vi "solar_cfg Read File (Var).vi"(0 "Config Path (*.ini)":path, 1 "Section (\"\" = Use Filename)":string, 2 "Comments (Key,Comment)":cluster{"Key":string, "Comment":string}[](array[cluster]), 5 "Key_Prefix (\"\")":string, 7 "Variant in":variant, 11 "error in (no error)":errorcluster, 12 "ArrayDelimiters (1D,2D)":string[](array[string]), 13 "Write If Not Found? (T)":bool=TRUE) -> (4 "Config Path out":path, 6 "Variant out":variant, 10 "Found?":bool, 15 "error out":errorcluster)   [LabVIEW 2018]
doc: "Reads the values associated with a variant from a specified section in a configuration file. If the Key is empty the variant label is used instead. Set a Comment (#...) to add a description after the key's value. Clusters use the element lables are their key names. Set Enum as Strings to True to use the string item of an enum.\n\nSupported Data Types: \nI8..EXT, Enum, Boolean, String, Path, VISA Reference, Timestamp\n1D & 2D Arrays and Clusters of the data types above.\n\n[Section]\nKey = \"Value\" #Comment"
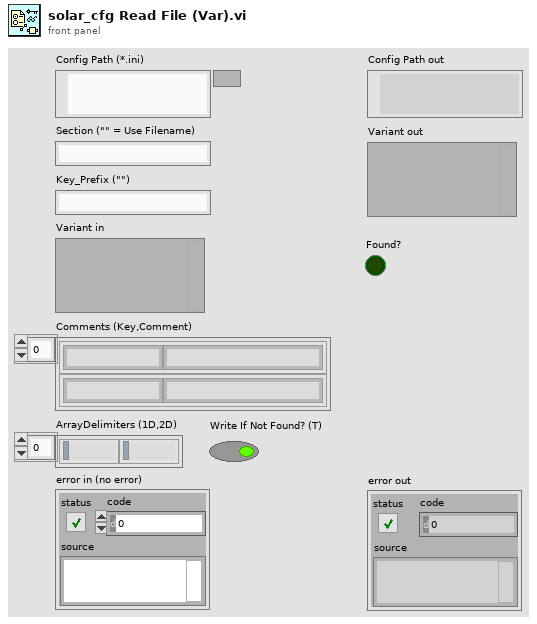
[diagram p1: front panel]
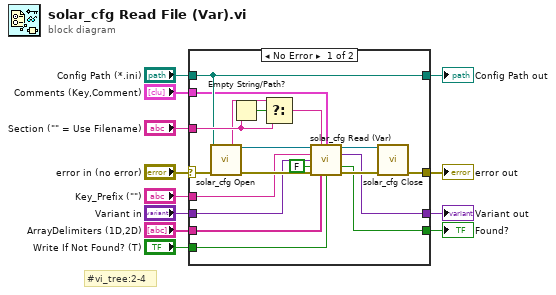
[diagram p0: block diagram]
diagram:
  # "#vi_tree:2-4"
  n1 = case shown="No Error" "error in (no error)" {
    selector: "error in (no error)" -> [w29 w34]
    tunnel: "Config Path (*.ini)" -> [w28 w33]
    tunnel: "Key_Prefix (\"\")" -> [w14 _]
    tunnel: [w18 w34] -> w9
    tunnel: "Section (\"\" = Use Filename)" -> [w30 _]
    tunnel: [w28 w33] -> w7
    tunnel: "Variant in" -> [w15 w32]
    tunnel: [w17 w32] -> w5
    tunnel: "Comments (Key,Comment)" -> [w24 _]
    tunnel: "ArrayDelimiters (1D,2D)" -> [w22 _]
    tunnel: "Write If Not Found? (T)" -> [w21 _]
    tunnel: [w16 _] -> w1
    frame No Error {
      n2 = call "solar_cfg Open.vi"("Config Path (*.ini)"=w28, "error in (no error)"=w29) -> ("Filename"=w27:string, "Config Refnum"=w23:refnum<data-value>, "error out"=w26:errorcluster)  [unwired: 10 in, 1 out]
      n3 = Empty String/Path?(string/path=w30) -> (empty?=w31:bool)
      n4 = Select(t=w27, s=w31, f=w30) -> (s? t:f=w25:string)
      n5 = call "solar_cfg Read (Var).vi"("Config Refnum"=w23, "Section"=w25, "Comments (Key,Comment)"=w24, "Key (\"\")"=w14, "Variant in"=w15, "Include Variant Name? (F)"=FALSE ("Include Prefix? (T)"), "error in (no error)"=w26, "ArrayDelimiters (1D,2D)"=w22, "Write If Not Found? (T)"=w21) -> ("dup Config Refnum"=w19:refnum<data-value>, "Variant out"=w17:variant, "Found?"=w16:bool, "error out"=w20:errorcluster)  [unwired: 3 in]
      n6 = call "solar_cfg Close.vi"("Config Refnum"=w19, "error in (no error)"=w20) -> ("error out"=w18:errorcluster)  [unwired: 12 in, 1 out]
    }
    frame Error {
    }
  }
  "error out" <- w9
  "Config Path out" <- w7
  "Variant out" <- w5
  "Found?" <- w1
